vi "LSMcontroller_v56_from here for labview64bit.vi"() -> ()   [LabVIEW 2015] (continued)
                    n4222 = Bundle By Name(cluster=w1106, "Drawing Mode"=w1079, "measpoints"=w1095, "tt_cycles"=w1097, "refreshbuffer"=w1092, "refreshrate"=w1091, "Vx-ref"=w1098, "Vy-ref"=w1100, "srate"=w1089, "finite"=w1102, "cont"=w1101, "wavdet"=w1103, "avpp"=w1099, "srateAODO"=w1096, "bufferAI"=w1092, "bin"=w1094, "Angle Img"=w1086, "Vxminref"=w1085, "Vxmaxref"=w1084, "Vyminref"=w1083, "Vymaxref"=w1082, "Xpixels Img"=w1081, "Ypixels Img"=w1080, "Pel"=w1078, "Vz-reset"=0.0, "AIoverride"=w1076, "type"="Lifetime (contour)") -> (w1104:T12)
                    n4223 = Reciprocal(x=w1091) -> (1/x=w1088:dbl)
                    n4224 = local write "refreshtime"(w1088) -> ()
                    n4225 = call "2pparameters.vi"("Params in"=w1104, "command"="set") -> ()  [unwired: 1 out]
                  }
                  frame "X-Y-Z-t movie" {
                  }
                  frame "linescan" {
                  }
                  frame "Timetrace" {
                    n4226 = local read "Vy-min draw"() -> (w1116:dbl)
                    n4227 = local read "Vy-max draw"() -> (w1115:dbl)
                    n4228 = local read "Vx-min draw"() -> (w1118:dbl)
                    n4229 = local read "Vx-max draw"() -> (w1117:dbl)
                    n4230 = local read "xpixels ref"() -> (w1114:i32)
                    n4231 = local read "ypixels ref"() -> (w1113:i32)
                    n4232 = local read "ROI Type"() -> (w1112:u16)
                    n4233 = local read "srateAODOtt"() -> (w1123:dbl)
                    n4234 = local read "# of frames"() -> (w1128:i32)
                    n4235 = local read "refreshtime"() -> (w1120:dbl)
                    n4236 = local read "Pel"() -> (w1111:dbl)
                    n4237 = local read "bin"() -> (w1126:dbl)
                    n4238 = local read "Override AI buffer"() -> (w1109:bool)
                    n4239 = local read "finite samples"() -> (w1135:bool)
                    n4240 = local read "srateAODOtt"() -> (w1122:dbl)
                    n4241 = local read "srateAODOtt"() -> (w1129:dbl)
                    n4242 = local read "continuous"() -> (w1134:bool)
                    n4243 = local read "Angle ref"() -> (w1119:dbl)
                    n4244 = local read "wavdet"() -> (w1136:bool)
                    n4245 = local read "Vx-ref"() -> (w1131:dbl)
                    n4246 = local read "Vy-ref"() -> (w1133:dbl)
                    n4247 = local read "avpp"() -> (w1132:i32)
                    n4248 = call "tt_timeandsamples.vi"("bin"=w1126, "refreshtime"=w1120, "srateAODOtt"=w1123, "tot#ofsamples"=w1128) -> ("refreshrate"=w1124:dbl, "refreshbuffer"=w1125:i32, "timetracecycles"=w1130:i32)  [unwired: 5 in]
                    n4249 = local read "bin"() -> (w1127:dbl)
                    n4250 = call "2pparameters.vi"("command"="get") -> ("params out"=w1139:T12)  [unwired: 1 in]
                    n4251 = Bundle By Name(cluster=w1139, "Drawing Mode"=w1112, "measpoints"=w1128, "tt_cycles"=w1130, "refreshbuffer"=w1125, "refreshrate"=w1124, "Vx-ref"=w1131, "Vy-ref"=w1133, "srate"=w1122, "finite"=w1135, "cont"=w1134, "wavdet"=w1136, "avpp"=w1132, "srateAODO"=w1129, "bufferAI"=w1125, "bin"=w1127, "Angle Img"=w1119, "Vxminref"=w1118, "Vxmaxref"=w1117, "Vyminref"=w1116, "Vymaxref"=w1115, "Xpixels Img"=w1114, "Ypixels Img"=w1113, "Pel"=w1111, "Vz-reset"=0.0, "AIoverride"=w1109, "type"="Timetrace") -> (w1137:T12)
                    n4252 = Reciprocal(x=w1124) -> (1/x=w1121:dbl)
                    n4253 = local write "refreshtime"(w1121) -> ()
                    n4254 = call "2pparameters.vi"("Params in"=w1137, "command"="set") -> ()  [unwired: 1 out]
                  }
                  frame "Lifetime (point)" {
                  }
                }
              }
              frame #1 {
                w1142 = FALSE ("wavdet")
                n4255 = call "2pparameters.vi"("command"="get") -> ("params out"=w1146:T12)  [unwired: 1 in]
                n4256 = Bundle By Name(cluster=w1146, "finite"=w1142, "cont"=w1142, "wavdet"=TRUE) -> (w1143:T12)
                n4257 = call "2pparameters.vi"("Params in"=w1143, "command"="set") -> ()  [unwired: 1 out]
              }
              frame #2 {
                n4258 = local read "Meastab"() -> (w1151:enum32{"X-Y Image", "Linescan", "Timetrace"})
                n4259 = property on="refwf" class="Ring (strict)"() -> ("RingText.Text"=w1154:string)  [unwired: 2 in, 2 out]
                n4260 = case shown="\"Timetrace\"" w1151 {
                  tunnel: [w1164 w1165] -> w1150
                  frame "X-Y Image", Default {
                    n4261 = local read "Sampling rate"() -> (w1164:dbl)
                  }
                  frame "Timetrace" {
                    n4262 = local read "srateAODOtt"() -> (w1165:dbl)
                  }
                }
                n4263 = call "waveformsAObuffer.vi"("command"="get") -> ("AO wf out"=w1163:waveform(dbl)[])  [unwired: 1 in]
                n4264 = local read "wavdet"() -> (w1153:bool)
                n4265 = call "waveformsDObuffer.vi"("command"="get") -> ("DO wf out"=w1159:digitalwaveform[])  [unwired: 1 in]
                n4266 = call "correctwaveformsizetemp.vi"("new sampling frequency (Hz)"=w1150, "start"=FALSE, "reference waveforms to"=w1154, "Analog waveforms in"=w1163, "stop"=FALSE, "Digital waveforms in"=w1159) -> ("analog wf out"=w1157:waveform(dbl)[], "Digital wf out"=w1155:digitalwaveform[], "measpoints"=w1152:i32)
                n4267 = local write "Analog Lines Plot"(w1157) -> ()
                n4268 = call "GetNumCamFramesv2.vi"("Digital Waveform Graph"=w1155) -> ("Numeric"=w1156:i32)  [unwired: 10 in]
                n4269 = local write "Digital Lines Plot"(w1155) -> ()
                n4270 = call "waveformsDObuffer.vi"("DO wf in"=w1155, "command"="set") -> ()  [unwired: 1 out]
                n4271 = call "waveformsAObuffer.vi"("AO wf in"=w1157, "command"="set") -> ()  [unwired: 1 out]
                n4272 = local write "Total Camera Frames"(w1156) -> ()
                n4273 = case shown="True" w1153 {
                  tunnel: w1152 -> [_ w1166]
                  frame False {
                  }
                  frame True {
                    n4274 = local write "# of frames"(w1166) -> ()
                  }
                }
              }
              frame #3 {
                n4275 = local read "finite samples"() -> (w1167:bool)
                n4276 = local read "continuous"() -> (w1168:bool)
                n4277 = local read "wavdet"() -> (w1169:bool)
                n4278 = call "2pparameters.vi"("command"="get") -> ("params out"=w1172:T12)  [unwired: 1 in]
                n4279 = Bundle By Name(cluster=w1172, "finite"=w1167, "cont"=w1168, "wavdet"=w1169) -> (w1170:T12)
                n4280 = call "2pparameters.vi"("Params in"=w1170, "command"="set") -> ()  [unwired: 1 out]
              }
            }
          }
          event "Start amplitude (V)", "Cycles", "Baseline (V)", "Step size (V)", "DC (%)", "Period (ms)", "Repeats", "Pulses", "phase shift (ms)": Value Change {
            n4281 = event-data() -> ()  [unwired: 1 in, 6 out]
            n4282 = stacked-sequence {
              seq-local: [_ _ w1280 _ _] -> [_ _ _ w1302 _]
              seq-local: [_ _ w1279 _ _] -> [_ _ _ w1301 _]
              frame #0 {
                n4283 = local read "Measurement"() -> (w1174:T5)
                n4284 = case shown="\"X-Y-t movie\", Default" w1174 {
                  frame "X-Y-t movie", Default {
                    n4285 = local read "avpp"() -> (w1195:i32)
                    n4286 = local read "Angle ref"() -> (w1194:dbl)
                    n4287 = local read "ROI Type"() -> (w1193:u16)
                    n4288 = local read "xpixels ref"() -> (w1190:i32)
                    n4289 = local read "Vx-min ref"() -> (w1189:dbl)
                    n4290 = local read "Vx-max ref"() -> (w1188:dbl)
                    n4291 = local read "ypixels ref"() -> (w1186:i32)
                    n4292 = local read "Vy-min ref"() -> (w1187:dbl)
                    n4293 = local read "Vy-max ref"() -> (w1183:dbl)
                    n4294 = local read "Sampling rate"() -> (w1177:dbl)
                    n4295 = local read "finite samples"() -> (w1178:bool)
                    n4296 = local read "continuous"() -> (w1181:bool)
                    n4297 = local read "wavdet"() -> (w1182:bool)
                    n4298 = local read "# of frames"() -> (w1180:i32)
                    n4299 = local read "maxbufferAI"() -> (w1179:i32)
                    n4300 = local read "Override AI buffer"() -> (w1175:bool)
                    n4301 = call "2pparameters.vi"("command"="get") -> ("params out"=w1192:T12)  [unwired: 1 in]
                    n4302 = Bundle By Name(cluster=w1192, "type"="X-Y-t movie", "avpp"=w1195, "Angle Img"=w1194, "Xpixels Img"=w1190, "Vx-min Img"=w1189, "VX-max Img"=w1188, "Ypixels Img"=w1186, "Vy-min Img"=w1187, "Vy-max Img"=w1183, "srate"=w1177, "srate Img"=w1177, "finite"=w1178, "cont"=w1181, "wavdet"=w1182, "measpoints"=w1180, "maxbufferAI"=w1179, "Drawing Mode"=w1193, "Vz-reset"=0.0, "AIoverride"=w1175) -> (w1184:T12)
                    n4303 = call "2pparameters.vi"("Params in"=w1184, "command"="set") -> ()  [unwired: 1 out]
                  }
                  frame "X-Y-Z stack" {
                    n4304 = call "2pparameters.vi"("command"="get") -> ("params out"=w1199:T12)  [unwired: 1 in]
                    n4305 = Bundle By Name(cluster=w1199, "type"="X-Y-Z stack") -> (w1197:T12)
                    n4306 = call "2pparameters.vi"("Params in"=w1197, "command"="set") -> ()  [unwired: 1 out]
                  }
                  frame "Lifetime (scan)" {
                    n4307 = call "2pparameters.vi"("command"="get") -> ("params out"=w1204:T12)  [unwired: 1 in]
                    n4308 = Bundle By Name(cluster=w1204, "type"="Lifetime (scan)") -> (w1202:T12)
                    n4309 = call "2pparameters.vi"("Params in"=w1202, "command"="set") -> ()  [unwired: 1 out]
                  }
                  frame "Lifetime (contour)" {
                    n4310 = local read "Vy-min draw"() -> (w1214:dbl)
                    n4311 = local read "Vy-max draw"() -> (w1213:dbl)
                    n4312 = local read "Vx-min draw"() -> (w1216:dbl)
                    n4313 = local read "Vx-max draw"() -> (w1215:dbl)
                    n4314 = local read "xpixels ref"() -> (w1212:i32)
                    n4315 = local read "ypixels ref"() -> (w1211:i32)
                    n4316 = local read "ROI Type"() -> (w1210:u16)
                    n4317 = local read "srateAODOtt"() -> (w1221:dbl)
                    n4318 = local read "# of frames"() -> (w1226:i32)
                    n4319 = local read "refreshtime"() -> (w1218:dbl)
                    n4320 = local read "Pel"() -> (w1209:dbl)
                    n4321 = local read "bin"() -> (w1224:dbl)
                    n4322 = local read "Override AI buffer"() -> (w1207:bool)
                    n4323 = local read "finite samples"() -> (w1233:bool)
                    n4324 = local read "srateAODOtt"() -> (w1220:dbl)
                    n4325 = local read "srateAODOtt"() -> (w1227:dbl)
                    n4326 = local read "continuous"() -> (w1232:bool)
                    n4327 = local read "Angle ref"() -> (w1217:dbl)
                    n4328 = local read "wavdet"() -> (w1234:bool)
                    n4329 = local read "Vx-ref"() -> (w1229:dbl)
                    n4330 = local read "Vy-ref"() -> (w1231:dbl)
                    n4331 = local read "avpp"() -> (w1230:i32)
                    n4332 = call "tt_timeandsamples.vi"("bin"=w1224, "refreshtime"=w1218, "srateAODOtt"=w1221, "tot#ofsamples"=w1226) -> ("refreshrate"=w1222:dbl, "refreshbuffer"=w1223:i32, "timetracecycles"=w1228:i32)  [unwired: 5 in]
                    n4333 = local read "bin"() -> (w1225:dbl)
                    n4334 = call "2pparameters.vi"("command"="get") -> ("params out"=w1237:T12)  [unwired: 1 in]
                    n4335 = Bundle By Name(cluster=w1237, "Drawing Mode"=w1210, "measpoints"=w1226, "tt_cycles"=w1228, "refreshbuffer"=w1223, "refreshrate"=w1222, "Vx-ref"=w1229, "Vy-ref"=w1231, "srate"=w1220, "finite"=w1233, "cont"=w1232, "wavdet"=w1234, "avpp"=w1230, "srateAODO"=w1227, "bufferAI"=w1223, "bin"=w1225, "Angle Img"=w1217, "Vxminref"=w1216, "Vxmaxref"=w1215, "Vyminref"=w1214, "Vymaxref"=w1213, "Xpixels Img"=w1212, "Ypixels Img"=w1211, "Pel"=w1209, "Vz-reset"=0.0, "AIoverride"=w1207, "type"="Lifetime (contour)") -> (w1235:T12)
                    n4336 = Reciprocal(x=w1222) -> (1/x=w1219:dbl)
                    n4337 = local write "refreshtime"(w1219) -> ()
                    n4338 = call "2pparameters.vi"("Params in"=w1235, "command"="set") -> ()  [unwired: 1 out]
                  }
                  frame "X-Y-Z-t movie" {
                  }
                  frame "linescan" {
                  }
                  frame "Timetrace" {
                    n4339 = local read "Vy-min draw"() -> (w1247:dbl)
                    n4340 = local read "Vy-max draw"() -> (w1246:dbl)
                    n4341 = local read "Vx-min draw"() -> (w1249:dbl)
                    n4342 = local read "Vx-max draw"() -> (w1248:dbl)
                    n4343 = local read "xpixels ref"() -> (w1245:i32)
                    n4344 = local read "ypixels ref"() -> (w1244:i32)
                    n4345 = local read "ROI Type"() -> (w1243:u16)
                    n4346 = local read "srateAODOtt"() -> (w1254:dbl)
                    n4347 = local read "# of frames"() -> (w1259:i32)
                    n4348 = local read "refreshtime"() -> (w1251:dbl)
                    n4349 = local read "Pel"() -> (w1242:dbl)
                    n4350 = local read "bin"() -> (w1257:dbl)
                    n4351 = local read "Override AI buffer"() -> (w1240:bool)
                    n4352 = local read "finite samples"() -> (w1266:bool)
                    n4353 = local read "srateAODOtt"() -> (w1253:dbl)
                    n4354 = local read "srateAODOtt"() -> (w1260:dbl)
                    n4355 = local read "continuous"() -> (w1265:bool)
                    n4356 = local read "Angle ref"() -> (w1250:dbl)
                    n4357 = local read "wavdet"() -> (w1267:bool)
                    n4358 = local read "Vx-ref"() -> (w1262:dbl)
                    n4359 = local read "Vy-ref"() -> (w1264:dbl)
                    n4360 = local read "avpp"() -> (w1263:i32)
                    n4361 = call "tt_timeandsamples.vi"("bin"=w1257, "refreshtime"=w1251, "srateAODOtt"=w1254, "tot#ofsamples"=w1259) -> ("refreshrate"=w1255:dbl, "refreshbuffer"=w1256:i32, "timetracecycles"=w1261:i32)  [unwired: 5 in]
                    n4362 = local read "bin"() -> (w1258:dbl)
                    n4363 = call "2pparameters.vi"("command"="get") -> ("params out"=w1270:T12)  [unwired: 1 in]
                    n4364 = Bundle By Name(cluster=w1270, "Drawing Mode"=w1243, "measpoints"=w1259, "tt_cycles"=w1261, "refreshbuffer"=w1256, "refreshrate"=w1255, "Vx-ref"=w1262, "Vy-ref"=w1264, "srate"=w1253, "finite"=w1266, "cont"=w1265, "wavdet"=w1267, "avpp"=w1263, "srateAODO"=w1260, "bufferAI"=w1256, "bin"=w1258, "Angle Img"=w1250, "Vxminref"=w1249, "Vxmaxref"=w1248, "Vyminref"=w1247, "Vymaxref"=w1246, "Xpixels Img"=w1245, "Ypixels Img"=w1244, "Pel"=w1242, "Vz-reset"=0.0, "AIoverride"=w1240, "type"="Timetrace") -> (w1268:T12)
                    n4365 = Reciprocal(x=w1255) -> (1/x=w1252:dbl)
                    n4366 = local write "refreshtime"(w1252) -> ()
                    n4367 = call "2pparameters.vi"("Params in"=w1268, "command"="set") -> ()  [unwired: 1 out]
                  }
                  frame "Lifetime (point)" {
                  }
                }
              }
              frame #1 {
                w1273 = FALSE ("wavdet")
                n4368 = call "2pparameters.vi"("command"="get") -> ("params out"=w1277:T12)  [unwired: 1 in]
                n4369 = Bundle By Name(cluster=w1277, "finite"=w1273, "cont"=w1273, "wavdet"=TRUE) -> (w1274:T12)
                n4370 = call "2pparameters.vi"("Params in"=w1274, "command"="set") -> ()  [unwired: 1 out]
              }
              frame #2 {
                n4371 = local read "AO channels"() -> (w1282:u32)
                n4372 = call "2pparameters.vi"("command"="get") -> ("params out"=w1284:T12)  [unwired: 1 in]
                n4373 = Unbundle By Name(w1284) -> ("aAO"=w1283:u32[])
                n4374 = Search 1D Array(1D array=w1283, element=w1282) -> (index of element=w1280:i32)  [unwired: 1 in]
                n4375 = Greater?(x=w1280, y=-1) -> (0:w1279:bool)
                n4376 = case shown="True" w1279 {
                  tunnel: w1280 -> [_ w1298]
                  frame False {
                  }
                  frame True {
                    n4377 = local read "Meastab"() -> (w1287:enum32{"X-Y Image", "Linescan", "Timetrace"})
                    n4378 = case shown="\"Timetrace\"" w1287 {
                      tunnel: [w1299 w1300] -> w1286
                      frame "X-Y Image", Default {
                        n4379 = local read "Sampling rate"() -> (w1299:dbl)
                      }
                      frame "Timetrace" {
                        n4380 = local read "srateAODOtt"() -> (w1300:dbl)
                      }
                    }
                    n4381 = local read "Start amplitude (V)"() -> (w1295:dbl)
                    n4382 = local read "phase shift (ms)"() -> (w1290:dbl)
                    n4383 = local read "Step size (V)"() -> (w1293:dbl)
                    n4384 = local read "Baseline (V)"() -> (w1294:dbl)
                    n4385 = local read "Period (ms)"() -> (w1291:dbl)
                    n4386 = local read "padding value"() -> (w1288:dbl)
                    n4387 = local read "Repeats"() -> (w1297:dbl)
                    n4388 = local read "Cycles"() -> (w1296:dbl)
                    n4389 = local read "DC (%)"() -> (w1292:dbl)
                    n4390 = local read "Pulses"() -> (w1289:dbl)
                    n4391 = call "replace AO square wf param.vi"("Baseline (V)"=w1294, "Start amplitude (V)"=w1295, "Cycles"=w1296, "Repeats"=w1297, "index of AO wave"=w1298, "Step size (V)"=w1293, "DC (%)"=w1292, "Sampling frequency (Hz)"=w1286, "Period (ms)"=w1291, "Cycle length (s)"=w1290, "Pulses"=w1289, "padding value"=w1288) -> ()  [unwired: 4 in]
                  }
                }
              }
              frame #3 {
                n4392 = case shown="True" w1301 {
                  tunnel: w1302 -> [_ w1310]
                  frame False {
                  }
                  frame True {
                    n4393 = call "waveformparamsv2.vi"("command"="get") -> ("Params out"=w1324:T16)  [unwired: 4 in, 2 out]
                    n4394 = Unbundle By Name(w1324) -> ("AO parameters"=w1323:T17)
                    n4395 = local read "Meastab"() -> (w1305:enum32{"X-Y Image", "Linescan", "Timetrace"})
                    n4396 = case shown="\"Timetrace\"" w1305 {
                      tunnel: [w1326 w1327] -> w1314
                      frame "X-Y Image", Default {
                        n4397 = local read "Sampling rate"() -> (w1326:dbl)
                      }
                      frame "Timetrace" {
                        n4398 = local read "srateAODOtt"() -> (w1327:dbl)
                      }
                    }
                    n4399 = Index Array(array=w1323, index=w1310) -> (element=w1312:T18)
                    n4400 = call "waveformsAObuffer.vi"("command"="get") -> ("AO wf out"=w1311:waveform(dbl)[])  [unwired: 1 in]
                    n4401 = call "generateRampedSquareWave_fromAOparameters.vi"("AO params"=w1312) -> ("Waveform"=w1309:waveform(dbl))  [unwired: 1 out]
                    n4402 = property on="refwf" class="Ring (strict)"() -> ("RingText.Text"=w1313:string)  [unwired: 2 in, 2 out]
                    n4403 = Replace Array Subset(array=w1311, new element=w1309, index=w1310) -> (w1308:waveform(dbl)[])
                    n4404 = call "waveformsDObuffer.vi"("command"="get") -> ("DO wf out"=w1319:digitalwaveform[])  [unwired: 1 in]
                    n4405 = call "correctwaveformsizetemp.vi"("new sampling frequency (Hz)"=w1314, "start"=FALSE, "reference waveforms to"=w1313, "Analog waveforms in"=w1308, "stop"=FALSE, "Digital waveforms in"=w1319) -> ("analog wf out"=w1317:waveform(dbl)[], "Digital wf out"=w1315:digitalwaveform[], "measpoints"=w1306:i32)
                    n4406 = local read "wavdet"() -> (w1307:bool)
                    n4407 = local write "Analog Lines Plot"(w1317) -> ()
                    n4408 = call "GetNumCamFramesv2.vi"("Digital Waveform Graph"=w1315) -> ("Numeric"=w1316:i32)  [unwired: 10 in]
                    n4409 = local write "Digital Lines Plot"(w1315) -> ()
                    n4410 = call "waveformsAObuffer.vi"("AO wf in"=w1317, "command"="set") -> ()  [unwired: 1 out]
                    n4411 = call "waveformsDObuffer.vi"("DO wf in"=w1315, "command"="set") -> ()  [unwired: 1 out]
                    n4412 = local write "Total Camera Frames"(w1316) -> ()
                    n4413 = case shown="True" w1307 {
                      tunnel: w1306 -> [_ w1328]
                      frame False {
                      }
                      frame True {
                        n4414 = local write "# of frames"(w1328) -> ()
                      }
                    }
                  }
                }
              }
              frame #4 {
                n4415 = local read "finite samples"() -> (w1329:bool)
                n4416 = local read "continuous"() -> (w1330:bool)
                n4417 = local read "wavdet"() -> (w1331:bool)
                n4418 = call "2pparameters.vi"("command"="get") -> ("params out"=w1334:T12)  [unwired: 1 in]
                n4419 = Bundle By Name(cluster=w1334, "finite"=w1329, "cont"=w1330, "wavdet"=w1331) -> (w1332:T12)
                n4420 = call "2pparameters.vi"("Params in"=w1332, "command"="set") -> ()  [unwired: 1 out]
              }
            }
          }
          event "Amplitude (V)", "Offset (V)", "Frequency", "Tri Repeats": Value Change {
            n4421 = event-data() -> ()  [unwired: 1 in, 6 out]
            n4422 = stacked-sequence {
              seq-local: [_ _ w1442 _ _] -> [_ _ _ w1460 _]
              seq-local: [_ _ w1441 _ _] -> [_ _ _ w1459 _]
              frame #0 {
                n4423 = local read "Measurement"() -> (w1336:T5)
                n4424 = case shown="\"X-Y-t movie\", Default" w1336 {
                  frame "X-Y-t movie", Default {
                    n4425 = local read "avpp"() -> (w1357:i32)
                    n4426 = local read "Angle ref"() -> (w1356:dbl)
                    n4427 = local read "ROI Type"() -> (w1355:u16)
                    n4428 = local read "xpixels ref"() -> (w1352:i32)
                    n4429 = local read "Vx-min ref"() -> (w1351:dbl)
                    n4430 = local read "Vx-max ref"() -> (w1350:dbl)
                    n4431 = local read "ypixels ref"() -> (w1348:i32)
                    n4432 = local read "Vy-min ref"() -> (w1349:dbl)
                    n4433 = local read "Vy-max ref"() -> (w1345:dbl)
                    n4434 = local read "Sampling rate"() -> (w1339:dbl)
                    n4435 = local read "finite samples"() -> (w1340:bool)
                    n4436 = local read "continuous"() -> (w1343:bool)
                    n4437 = local read "wavdet"() -> (w1344:bool)
                    n4438 = local read "# of frames"() -> (w1342:i32)
                    n4439 = local read "maxbufferAI"() -> (w1341:i32)
                    n4440 = local read "Override AI buffer"() -> (w1337:bool)
                    n4441 = call "2pparameters.vi"("command"="get") -> ("params out"=w1354:T12)  [unwired: 1 in]
                    n4442 = Bundle By Name(cluster=w1354, "type"="X-Y-t movie", "avpp"=w1357, "Angle Img"=w1356, "Xpixels Img"=w1352, "Vx-min Img"=w1351, "VX-max Img"=w1350, "Ypixels Img"=w1348, "Vy-min Img"=w1349, "Vy-max Img"=w1345, "srate"=w1339, "srate Img"=w1339, "finite"=w1340, "cont"=w1343, "wavdet"=w1344, "measpoints"=w1342, "maxbufferAI"=w1341, "Drawing Mode"=w1355, "Vz-reset"=0.0, "AIoverride"=w1337) -> (w1346:T12)
                    n4443 = call "2pparameters.vi"("Params in"=w1346, "command"="set") -> ()  [unwired: 1 out]
                  }
                  frame "X-Y-Z stack" {
                    n4444 = call "2pparameters.vi"("command"="get") -> ("params out"=w1361:T12)  [unwired: 1 in]
                    n4445 = Bundle By Name(cluster=w1361, "type"="X-Y-Z stack") -> (w1359:T12)
                    n4446 = call "2pparameters.vi"("Params in"=w1359, "command"="set") -> ()  [unwired: 1 out]
                  }
                  frame "Lifetime (scan)" {
                    n4447 = call "2pparameters.vi"("command"="get") -> ("params out"=w1366:T12)  [unwired: 1 in]
                    n4448 = Bundle By Name(cluster=w1366, "type"="Lifetime (scan)") -> (w1364:T12)
                    n4449 = call "2pparameters.vi"("Params in"=w1364, "command"="set") -> ()  [unwired: 1 out]
                  }
                  frame "Lifetime (contour)" {
                    n4450 = local read "Vy-min draw"() -> (w1376:dbl)
                    n4451 = local read "Vy-max draw"() -> (w1375:dbl)
                    n4452 = local read "Vx-min draw"() -> (w1378:dbl)
                    n4453 = local read "Vx-max draw"() -> (w1377:dbl)
                    n4454 = local read "xpixels ref"() -> (w1374:i32)
                    n4455 = local read "ypixels ref"() -> (w1373:i32)
                    n4456 = local read "ROI Type"() -> (w1372:u16)
                    n4457 = local read "srateAODOtt"() -> (w1383:dbl)
                    n4458 = local read "# of frames"() -> (w1388:i32)
                    n4459 = local read "refreshtime"() -> (w1380:dbl)
                    n4460 = local read "Pel"() -> (w1371:dbl)
                    n4461 = local read "bin"() -> (w1386:dbl)
                    n4462 = local read "Override AI buffer"() -> (w1369:bool)
                    n4463 = local read "finite samples"() -> (w1395:bool)
                    n4464 = local read "srateAODOtt"() -> (w1382:dbl)
                    n4465 = local read "srateAODOtt"() -> (w1389:dbl)
                    n4466 = local read "continuous"() -> (w1394:bool)
                    n4467 = local read "Angle ref"() -> (w1379:dbl)
                    n4468 = local read "wavdet"() -> (w1396:bool)
                    n4469 = local read "Vx-ref"() -> (w1391:dbl)
                    n4470 = local read "Vy-ref"() -> (w1393:dbl)
                    n4471 = local read "avpp"() -> (w1392:i32)
                    n4472 = call "tt_timeandsamples.vi"("bin"=w1386, "refreshtime"=w1380, "srateAODOtt"=w1383, "tot#ofsamples"=w1388) -> ("refreshrate"=w1384:dbl, "refreshbuffer"=w1385:i32, "timetracecycles"=w1390:i32)  [unwired: 5 in]
                    n4473 = local read "bin"() -> (w1387:dbl)
                    n4474 = call "2pparameters.vi"("command"="get") -> ("params out"=w1399:T12)  [unwired: 1 in]
                    n4475 = Bundle By Name(cluster=w1399, "Drawing Mode"=w1372, "measpoints"=w1388, "tt_cycles"=w1390, "refreshbuffer"=w1385, "refreshrate"=w1384, "Vx-ref"=w1391, "Vy-ref"=w1393, "srate"=w1382, "finite"=w1395, "cont"=w1394, "wavdet"=w1396, "avpp"=w1392, "srateAODO"=w1389, "bufferAI"=w1385, "bin"=w1387, "Angle Img"=w1379, "Vxminref"=w1378, "Vxmaxref"=w1377, "Vyminref"=w1376, "Vymaxref"=w1375, "Xpixels Img"=w1374, "Ypixels Img"=w1373, "Pel"=w1371, "Vz-reset"=0.0, "AIoverride"=w1369, "type"="Lifetime (contour)") -> (w1397:T12)
                    n4476 = Reciprocal(x=w1384) -> (1/x=w1381:dbl)
                    n4477 = local write "refreshtime"(w1381) -> ()
                    n4478 = call "2pparameters.vi"("Params in"=w1397, "command"="set") -> ()  [unwired: 1 out]
                  }
                  frame "X-Y-Z-t movie" {
                  }
                  frame "linescan" {
                  }
                  frame "Timetrace" {
                    n4479 = local read "Vy-min draw"() -> (w1409:dbl)
                    n4480 = local read "Vy-max draw"() -> (w1408:dbl)
                    n4481 = local read "Vx-min draw"() -> (w1411:dbl)
                    n4482 = local read "Vx-max draw"() -> (w1410:dbl)
                    n4483 = local read "xpixels ref"() -> (w1407:i32)
                    n4484 = local read "ypixels ref"() -> (w1406:i32)
                    n4485 = local read "ROI Type"() -> (w1405:u16)
                    n4486 = local read "srateAODOtt"() -> (w1416:dbl)
                    n4487 = local read "# of frames"() -> (w1421:i32)
                    n4488 = local read "refreshtime"() -> (w1413:dbl)
                    n4489 = local read "Pel"() -> (w1404:dbl)
                    n4490 = local read "bin"() -> (w1419:dbl)
                    n4491 = local read "Override AI buffer"() -> (w1402:bool)
                    n4492 = local read "finite samples"() -> (w1428:bool)
                    n4493 = local read "srateAODOtt"() -> (w1415:dbl)
                    n4494 = local read "srateAODOtt"() -> (w1422:dbl)
                    n4495 = local read "continuous"() -> (w1427:bool)
                    n4496 = local read "Angle ref"() -> (w1412:dbl)
                    n4497 = local read "wavdet"() -> (w1429:bool)
                    n4498 = local read "Vx-ref"() -> (w1424:dbl)
                    n4499 = local read "Vy-ref"() -> (w1426:dbl)
                    n4500 = local read "avpp"() -> (w1425:i32)
                    n4501 = call "tt_timeandsamples.vi"("bin"=w1419, "refreshtime"=w1413, "srateAODOtt"=w1416, "tot#ofsamples"=w1421) -> ("refreshrate"=w1417:dbl, "refreshbuffer"=w1418:i32, "timetracecycles"=w1423:i32)  [unwired: 5 in]
                    n4502 = local read "bin"() -> (w1420:dbl)
                    n4503 = call "2pparameters.vi"("command"="get") -> ("params out"=w1432:T12)  [unwired: 1 in]
                    n4504 = Bundle By Name(cluster=w1432, "Drawing Mode"=w1405, "measpoints"=w1421, "tt_cycles"=w1423, "refreshbuffer"=w1418, "refreshrate"=w1417, "Vx-ref"=w1424, "Vy-ref"=w1426, "srate"=w1415, "finite"=w1428, "cont"=w1427, "wavdet"=w1429, "avpp"=w1425, "srateAODO"=w1422, "bufferAI"=w1418, "bin"=w1420, "Angle Img"=w1412, "Vxminref"=w1411, "Vxmaxref"=w1410, "Vyminref"=w1409, "Vymaxref"=w1408, "Xpixels Img"=w1407, "Ypixels Img"=w1406, "Pel"=w1404, "Vz-reset"=0.0, "AIoverride"=w1402, "type"="Timetrace") -> (w1430:T12)
                    n4505 = Reciprocal(x=w1417) -> (1/x=w1414:dbl)
                    n4506 = local write "refreshtime"(w1414) -> ()
                    n4507 = call "2pparameters.vi"("Params in"=w1430, "command"="set") -> ()  [unwired: 1 out]
                  }
                  frame "Lifetime (point)" {
                  }
                }
              }
              frame #1 {
                w1435 = FALSE ("wavdet")
                n4508 = call "2pparameters.vi"("command"="get") -> ("params out"=w1439:T12)  [unwired: 1 in]
                n4509 = Bundle By Name(cluster=w1439, "finite"=w1435, "cont"=w1435, "wavdet"=TRUE) -> (w1436:T12)
                n4510 = call "2pparameters.vi"("Params in"=w1436, "command"="set") -> ()  [unwired: 1 out]
              }
              frame #2 {
                n4511 = local read "AO channels"() -> (w1444:u32)
                n4512 = call "2pparameters.vi"("command"="get") -> ("params out"=w1446:T12)  [unwired: 1 in]
                n4513 = Unbundle By Name(w1446) -> ("aAO"=w1445:u32[])
                n4514 = Search 1D Array(1D array=w1445, element=w1444) -> (index of element=w1442:i32)  [unwired: 1 in]
                n4515 = Greater?(x=w1442, y=-1) -> (0:w1441:bool)
                n4516 = case shown="True" w1441 {
                  tunnel: w1442 -> [_ w1456]
                  frame False {
                  }
                  frame True {
                    n4517 = local read "Meastab"() -> (w1449:enum32{"X-Y Image", "Linescan", "Timetrace"})
                    n4518 = local read "Tri padding value"() -> (w1450:dbl)
                    n4519 = local read "Amplitude (V)"() -> (w1454:dbl)
                    n4520 = local read "Tri Phase (s)"() -> (w1451:dbl)
                    n4521 = local read "Tri Repeats"() -> (w1452:dbl)
                    n4522 = local read "Frequency"() -> (w1453:dbl)
                    n4523 = local read "Offset (V)"() -> (w1455:dbl)
                    n4524 = case shown="\"Timetrace\"" w1449 {
                      tunnel: [w1457 w1458] -> w1448
                      frame "X-Y Image", Default {
                        n4525 = local read "Sampling rate"() -> (w1457:dbl)
                      }
                      frame "Timetrace" {
                        n4526 = local read "srateAODOtt"() -> (w1458:dbl)
                      }
                    }
                    n4527 = call "replace AO tri wf param.vi"("padding value"=w1450, "index of AO wave"=w1456, "Tri phase"=w1451, "Sampling frequency (Hz)"=w1448, "Tri Repeats"=w1452, "Frequency"=w1453, "Amplitude (V)"=w1454, "Offset (V)"=w1455) -> ()
                  }
                }
              }
              frame #3 {
                n4528 = case shown="True" w1459 {
                  tunnel: w1460 -> [_ w1469]
                  frame False {
                  }
                  frame True {
                    n4529 = call "waveformparamsv2.vi"("command"="get") -> ("Params out"=w1482:T16)  [unwired: 4 in, 2 out]
                    n4530 = Unbundle By Name(w1482) -> ("AO parameters"=w1481:T17)
                    n4531 = local read "Meastab"() -> (w1464:enum32{"X-Y Image", "Linescan", "Timetrace"})
                    n4532 = case shown="\"Timetrace\"" w1464 {
                      tunnel: [w1484 w1485] -> w1463
                      frame "X-Y Image", Default {
                        n4533 = local read "Sampling rate"() -> (w1484:dbl)
                      }
                      frame "Timetrace" {
                        n4534 = local read "srateAODOtt"() -> (w1485:dbl)
                      }
                    }
                    n4535 = Index Array(array=w1481, index=w1469) -> (element=w1471:T18)
                    n4536 = call "waveformsAObuffer.vi"("command"="get") -> ("AO wf out"=w1470:waveform(dbl)[])  [unwired: 1 in]
                    n4537 = call "generateTriWave_fromAOparameters.vi"("AO params"=w1471) -> ("Waveform"=w1468:waveform(dbl))  [unwired: 1 out]
                    n4538 = property on="refwf" class="Ring (strict)"() -> ("RingText.Text"=w1472:string)  [unwired: 2 in, 2 out]
                    n4539 = Replace Array Subset(array=w1470, new element=w1468, index=w1469) -> (w1467:waveform(dbl)[])
                    n4540 = call "waveformsDObuffer.vi"("command"="get") -> ("DO wf out"=w1477:digitalwaveform[])  [unwired: 1 in]
                    n4541 = call "correctwaveformsizetemp.vi"("new sampling frequency (Hz)"=w1463, "start"=FALSE, "reference waveforms to"=w1472, "Analog waveforms in"=w1467, "stop"=FALSE, "Digital waveforms in"=w1477) -> ("analog wf out"=w1475:waveform(dbl)[], "Digital wf out"=w1473:digitalwaveform[], "measpoints"=w1465:i32)
                    n4542 = local read "wavdet"() -> (w1466:bool)
                    n4543 = local write "Analog Lines Plot"(w1475) -> ()
                    n4544 = call "GetNumCamFramesv2.vi"("Digital Waveform Graph"=w1473) -> ("Numeric"=w1474:i32)  [unwired: 10 in]
                    n4545 = local write "Digital Lines Plot"(w1473) -> ()
                    n4546 = call "waveformsAObuffer.vi"("AO wf in"=w1475, "command"="set") -> ()  [unwired: 1 out]
                    n4547 = call "waveformsDObuffer.vi"("DO wf in"=w1473, "command"="set") -> ()  [unwired: 1 out]
                    n4548 = local write "Total Camera Frames"(w1474) -> ()
                    n4549 = case shown="True" w1466 {
                      tunnel: w1465 -> [_ w1486]
                      frame False {
                      }
                      frame True {
                        n4550 = local write "# of frames"(w1486) -> ()
                      }
                    }
                  }
                }
              }
              frame #4 {
                n4551 = local read "finite samples"() -> (w1487:bool)
                n4552 = local read "continuous"() -> (w1488:bool)
                n4553 = local read "wavdet"() -> (w1489:bool)
                n4554 = call "2pparameters.vi"("command"="get") -> ("params out"=w1492:T12)  [unwired: 1 in]
                n4555 = Bundle By Name(cluster=w1492, "finite"=w1487, "cont"=w1488, "wavdet"=w1489) -> (w1490:T12)
                n4556 = call "2pparameters.vi"("Params in"=w1490, "command"="set") -> ()  [unwired: 1 out]
              }
            }
          }
          event "Load Matlab Waveform": Value Change {
            n4557 = event-data() -> ()  [unwired: 1 in, 6 out]
            n4558 = stacked-sequence {
              seq-local: [_ _ w1600 _ _] -> [_ _ _ w1615 _]
              seq-local: [_ _ w1599 _ _] -> [_ _ _ w1614 _]
              frame #0 {
                n4559 = local read "Measurement"() -> (w1494:T5)
                n4560 = case shown="\"X-Y-t movie\", Default" w1494 {
                  frame "X-Y-t movie", Default {
                    n4561 = local read "avpp"() -> (w1515:i32)
                    n4562 = local read "Angle ref"() -> (w1514:dbl)
                    n4563 = local read "ROI Type"() -> (w1513:u16)
                    n4564 = local read "xpixels ref"() -> (w1510:i32)
                    n4565 = local read "Vx-min ref"() -> (w1509:dbl)
                    n4566 = local read "Vx-max ref"() -> (w1508:dbl)
                    n4567 = local read "ypixels ref"() -> (w1506:i32)
                    n4568 = local read "Vy-min ref"() -> (w1507:dbl)
                    n4569 = local read "Vy-max ref"() -> (w1503:dbl)
                    n4570 = local read "Sampling rate"() -> (w1497:dbl)
                    n4571 = local read "finite samples"() -> (w1498:bool)
                    n4572 = local read "continuous"() -> (w1501:bool)
                    n4573 = local read "wavdet"() -> (w1502:bool)
                    n4574 = local read "# of frames"() -> (w1500:i32)
                    n4575 = local read "maxbufferAI"() -> (w1499:i32)
                    n4576 = local read "Override AI buffer"() -> (w1495:bool)
                    n4577 = call "2pparameters.vi"("command"="get") -> ("params out"=w1512:T12)  [unwired: 1 in]
                    n4578 = Bundle By Name(cluster=w1512, "type"="X-Y-t movie", "avpp"=w1515, "Angle Img"=w1514, "Xpixels Img"=w1510, "Vx-min Img"=w1509, "VX-max Img"=w1508, "Ypixels Img"=w1506, "Vy-min Img"=w1507, "Vy-max Img"=w1503, "srate"=w1497, "srate Img"=w1497, "finite"=w1498, "cont"=w1501, "wavdet"=w1502, "measpoints"=w1500, "maxbufferAI"=w1499, "Drawing Mode"=w1513, "Vz-reset"=0.0, "AIoverride"=w1495) -> (w1504:T12)
                    n4579 = call "2pparameters.vi"("Params in"=w1504, "command"="set") -> ()  [unwired: 1 out]
                  }
                  frame "X-Y-Z stack" {
                    n4580 = call "2pparameters.vi"("command"="get") -> ("params out"=w1519:T12)  [unwired: 1 in]
                    n4581 = Bundle By Name(cluster=w1519, "type"="X-Y-Z stack") -> (w1517:T12)
                    n4582 = call "2pparameters.vi"("Params in"=w1517, "command"="set") -> ()  [unwired: 1 out]
                  }
                  frame "Lifetime (scan)" {
                    n4583 = call "2pparameters.vi"("command"="get") -> ("params out"=w1524:T12)  [unwired: 1 in]
                    n4584 = Bundle By Name(cluster=w1524, "type"="Lifetime (scan)") -> (w1522:T12)
                    n4585 = call "2pparameters.vi"("Params in"=w1522, "command"="set") -> ()  [unwired: 1 out]
                  }
                  frame "Lifetime (contour)" {
                    n4586 = local read "Vy-min draw"() -> (w1534:dbl)
                    n4587 = local read "Vy-max draw"() -> (w1533:dbl)
                    n4588 = local read "Vx-min draw"() -> (w1536:dbl)
                    n4589 = local read "Vx-max draw"() -> (w1535:dbl)
                    n4590 = local read "xpixels ref"() -> (w1532:i32)
                    n4591 = local read "ypixels ref"() -> (w1531:i32)
                    n4592 = local read "ROI Type"() -> (w1530:u16)
                    n4593 = local read "srateAODOtt"() -> (w1541:dbl)
                    n4594 = local read "# of frames"() -> (w1546:i32)
                    n4595 = local read "refreshtime"() -> (w1538:dbl)
                    n4596 = local read "Pel"() -> (w1529:dbl)
                    n4597 = local read "bin"() -> (w1544:dbl)
                    n4598 = local read "Override AI buffer"() -> (w1527:bool)
                    n4599 = local read "finite samples"() -> (w1553:bool)
                    n4600 = local read "srateAODOtt"() -> (w1540:dbl)
                    n4601 = local read "srateAODOtt"() -> (w1547:dbl)
                    n4602 = local read "continuous"() -> (w1552:bool)
                    n4603 = local read "Angle ref"() -> (w1537:dbl)
                    n4604 = local read "wavdet"() -> (w1554:bool)
                    n4605 = local read "Vx-ref"() -> (w1549:dbl)
                    n4606 = local read "Vy-ref"() -> (w1551:dbl)
                    n4607 = local read "avpp"() -> (w1550:i32)
                    n4608 = call "tt_timeandsamples.vi"("bin"=w1544, "refreshtime"=w1538, "srateAODOtt"=w1541, "tot#ofsamples"=w1546) -> ("refreshrate"=w1542:dbl, "refreshbuffer"=w1543:i32, "timetracecycles"=w1548:i32)  [unwired: 5 in]
                    n4609 = local read "bin"() -> (w1545:dbl)
                    n4610 = call "2pparameters.vi"("command"="get") -> ("params out"=w1557:T12)  [unwired: 1 in]
                    n4611 = Bundle By Name(cluster=w1557, "Drawing Mode"=w1530, "measpoints"=w1546, "tt_cycles"=w1548, "refreshbuffer"=w1543, "refreshrate"=w1542, "Vx-ref"=w1549, "Vy-ref"=w1551, "srate"=w1540, "finite"=w1553, "cont"=w1552, "wavdet"=w1554, "avpp"=w1550, "srateAODO"=w1547, "bufferAI"=w1543, "bin"=w1545, "Angle Img"=w1537, "Vxminref"=w1536, "Vxmaxref"=w1535, "Vyminref"=w1534, "Vymaxref"=w1533, "Xpixels Img"=w1532, "Ypixels Img"=w1531, "Pel"=w1529, "Vz-reset"=0.0, "AIoverride"=w1527, "type"="Lifetime (contour)") -> (w1555:T12)
                    n4612 = Reciprocal(x=w1542) -> (1/x=w1539:dbl)
                    n4613 = local write "refreshtime"(w1539) -> ()
                    n4614 = call "2pparameters.vi"("Params in"=w1555, "command"="set") -> ()  [unwired: 1 out]
                  }
                  frame "X-Y-Z-t movie" {
                  }
                  frame "linescan" {
                  }
                  frame "Timetrace" {
                    n4615 = local read "Vy-min draw"() -> (w1567:dbl)
                    n4616 = local read "Vy-max draw"() -> (w1566:dbl)
                    n4617 = local read "Vx-min draw"() -> (w1569:dbl)
                    n4618 = local read "Vx-max draw"() -> (w1568:dbl)
                    n4619 = local read "xpixels ref"() -> (w1565:i32)
                    n4620 = local read "ypixels ref"() -> (w1564:i32)
                    n4621 = local read "ROI Type"() -> (w1563:u16)
                    n4622 = local read "srateAODOtt"() -> (w1574:dbl)
                    n4623 = local read "# of frames"() -> (w1579:i32)
                    n4624 = local read "refreshtime"() -> (w1571:dbl)
                    n4625 = local read "Pel"() -> (w1562:dbl)
                    n4626 = local read "bin"() -> (w1577:dbl)
                    n4627 = local read "Override AI buffer"() -> (w1560:bool)
                    n4628 = local read "finite samples"() -> (w1586:bool)
                    n4629 = local read "srateAODOtt"() -> (w1573:dbl)
                    n4630 = local read "srateAODOtt"() -> (w1580:dbl)
                    n4631 = local read "continuous"() -> (w1585:bool)
                    n4632 = local read "Angle ref"() -> (w1570:dbl)
                    n4633 = local read "wavdet"() -> (w1587:bool)
                    n4634 = local read "Vx-ref"() -> (w1582:dbl)
                    n4635 = local read "Vy-ref"() -> (w1584:dbl)
                    n4636 = local read "avpp"() -> (w1583:i32)
                    n4637 = call "tt_timeandsamples.vi"("bin"=w1577, "refreshtime"=w1571, "srateAODOtt"=w1574, "tot#ofsamples"=w1579) -> ("refreshrate"=w1575:dbl, "refreshbuffer"=w1576:i32, "timetracecycles"=w1581:i32)  [unwired: 5 in]
                    n4638 = local read "bin"() -> (w1578:dbl)
                    n4639 = call "2pparameters.vi"("command"="get") -> ("params out"=w1590:T12)  [unwired: 1 in]
                    n4640 = Bundle By Name(cluster=w1590, "Drawing Mode"=w1563, "measpoints"=w1579, "tt_cycles"=w1581, "refreshbuffer"=w1576, "refreshrate"=w1575, "Vx-ref"=w1582, "Vy-ref"=w1584, "srate"=w1573, "finite"=w1586, "cont"=w1585, "wavdet"=w1587, "avpp"=w1583, "srateAODO"=w1580, "bufferAI"=w1576, "bin"=w1578, "Angle Img"=w1570, "Vxminref"=w1569, "Vxmaxref"=w1568, "Vyminref"=w1567, "Vymaxref"=w1566, "Xpixels Img"=w1565, "Ypixels Img"=w1564, "Pel"=w1562, "Vz-reset"=0.0, "AIoverride"=w1560, "type"="Timetrace") -> (w1588:T12)
                    n4641 = Reciprocal(x=w1575) -> (1/x=w1572:dbl)
                    n4642 = local write "refreshtime"(w1572) -> ()
                    n4643 = call "2pparameters.vi"("Params in"=w1588, "command"="set") -> ()  [unwired: 1 out]
                  }
                  frame "Lifetime (point)" {
                  }
                }
              }
              frame #1 {
                w1593 = FALSE ("wavdet")
                n4644 = call "2pparameters.vi"("command"="get") -> ("params out"=w1597:T12)  [unwired: 1 in]
                n4645 = Bundle By Name(cluster=w1597, "finite"=w1593, "cont"=w1593, "wavdet"=TRUE) -> (w1594:T12)
                n4646 = call "2pparameters.vi"("Params in"=w1594, "command"="set") -> ()  [unwired: 1 out]
              }
              frame #2 {
                n4647 = local read "AO channels"() -> (w1602:u32)
                n4648 = call "2pparameters.vi"("command"="get") -> ("params out"=w1604:T12)  [unwired: 1 in]
                n4649 = Unbundle By Name(w1604) -> ("aAO"=w1603:u32[])
                n4650 = Search 1D Array(1D array=w1603, element=w1602) -> (index of element=w1600:i32)  [unwired: 1 in]
                n4651 = Greater?(x=w1600, y=-1) -> (0:w1599:bool)
                n4652 = case shown="True" w1599 {
                  tunnel: w1600 -> [_ w1611]
                  frame False {
                  }
                  frame True {
                    n4653 = local read "Meastab"() -> (w1607:enum32{"X-Y Image", "Linescan", "Timetrace"})
                    n4654 = local read "Matlab waveform path"() -> (w1609:path)
                    n4655 = local read "Matlab padding value"() -> (w1610:dbl)
                    n4656 = case shown="\"Timetrace\"" w1607 {
                      tunnel: [w1612 w1613] -> w1606
                      frame "X-Y Image", Default {
                        n4657 = local read "Sampling rate"() -> (w1612:dbl)
                      }
                      frame "Timetrace" {
                        n4658 = local read "srateAODOtt"() -> (w1613:dbl)
                      }
                    }
                    n4659 = call "matlabwfexistsdialogue.vi"("Matlab waveform path"=w1609) -> ("mtalab waveform path out"=w1608:path)
                    n4660 = call "replace AO matlab param.vi"("Sampling frequency (Hz)"=w1606, "matlab wave file"=w1608, "index of AO wave"=w1611, "padding value"=w1610) -> ()  [unwired: 7 in]
                  }
                }
              }
              frame #3 {
                n4661 = case shown="True" w1614 {
                  tunnel: w1615 -> [_ w1622]
                  frame False {
                  }
                  frame True {
                    n4662 = local read "Meastab"() -> (w1619:enum32{"X-Y Image", "Linescan", "Timetrace"})
                    n4663 = call "waveformparamsv2.vi"("command"="get") -> ("Params out"=w1625:T16)  [unwired: 4 in, 2 out]
                    n4664 = Unbundle By Name(w1625) -> ("AO parameters"=w1624:T17)
                    n4665 = case shown="\"Timetrace\"" w1619 {
                      tunnel: [w1639 w1640] -> w1618
                      frame "X-Y Image", Default {
                        n4666 = local read "Sampling rate"() -> (w1639:dbl)
                      }
                      frame "Timetrace" {
                        n4667 = local read "srateAODOtt"() -> (w1640:dbl)
                      }
                    }
                    n4668 = Index Array(array=w1624, index=w1622) -> (element=w1623:T18)
                    n4669 = call "waveformsAObuffer.vi"("command"="get") -> ("AO wf out"=w1629:waveform(dbl)[])  [unwired: 1 in]
                    n4670 = call "matlabAOwffromparam.vi"("Cluster"=w1623) -> ("Waveform"=w1627:waveform(dbl))  [unwired: 1 out]
                    n4671 = property on="refwf" class="Ring (strict)"() -> ("RingText.Text"=w1630:string)  [unwired: 2 in, 2 out]
                    n4672 = Replace Array Subset(array=w1629, new element=w1627, index=w1622) -> (w1628:waveform(dbl)[])
                    n4673 = call "waveformsDObuffer.vi"("command"="get") -> ("DO wf out"=w1635:digitalwaveform[])  [unwired: 1 in]
                    n4674 = call "correctwaveformsizetemp.vi"("new sampling frequency (Hz)"=w1618, "start"=FALSE, "reference waveforms to"=w1630, "Analog waveforms in"=w1628, "stop"=FALSE, "Digital waveforms in"=w1635) -> ("analog wf out"=w1633:waveform(dbl)[], "Digital wf out"=w1631:digitalwaveform[], "measpoints"=w1620:i32)
                    n4675 = local read "wavdet"() -> (w1621:bool)
                    n4676 = local write "Analog Lines Plot"(w1633) -> ()
                    n4677 = call "GetNumCamFramesv2.vi"("Digital Waveform Graph"=w1631) -> ("Numeric"=w1632:i32)  [unwired: 10 in]
                    n4678 = local write "Digital Lines Plot"(w1631) -> ()
                    n4679 = call "waveformsAObuffer.vi"("AO wf in"=w1633, "command"="set") -> ()  [unwired: 1 out]
                    n4680 = call "waveformsDObuffer.vi"("DO wf in"=w1631, "command"="set") -> ()  [unwired: 1 out]
                    n4681 = local write "Total Camera Frames"(w1632) -> ()
                    n4682 = case shown="True" w1621 {
                      tunnel: w1620 -> [_ w1641]
                      frame False {
                      }
                      frame True {
                        n4683 = local write "# of frames"(w1641) -> ()
                      }
                    }
                  }
                }
              }
              frame #4 {
                n4684 = local read "finite samples"() -> (w1642:bool)
                n4685 = local read "continuous"() -> (w1643:bool)
                n4686 = local read "wavdet"() -> (w1644:bool)
                n4687 = call "2pparameters.vi"("command"="get") -> ("params out"=w1647:T12)  [unwired: 1 in]
                n4688 = Bundle By Name(cluster=w1647, "finite"=w1642, "cont"=w1643, "wavdet"=w1644) -> (w1645:T12)
                n4689 = call "2pparameters.vi"("Params in"=w1645, "command"="set") -> ()  [unwired: 1 out]
              }
            }
          }
          event "Load Matlab Waveform DO": Value Change {
            n4690 = event-data() -> ()  [unwired: 1 in, 6 out]
            n4691 = stacked-sequence {
              seq-local: [_ _ w1755 _ _] -> [_ _ _ w1770 _]
              seq-local: [_ _ w1754 _ _] -> [_ _ _ w1769 _]
              frame #0 {
                n4692 = local read "Measurement"() -> (w1649:T5)
                n4693 = case shown="\"X-Y-t movie\", Default" w1649 {
                  frame "X-Y-t movie", Default {
                    n4694 = local read "avpp"() -> (w1670:i32)
                    n4695 = local read "Angle ref"() -> (w1669:dbl)
                    n4696 = local read "ROI Type"() -> (w1668:u16)
                    n4697 = local read "xpixels ref"() -> (w1665:i32)
                    n4698 = local read "Vx-min ref"() -> (w1664:dbl)
                    n4699 = local read "Vx-max ref"() -> (w1663:dbl)
                    n4700 = local read "ypixels ref"() -> (w1661:i32)
                    n4701 = local read "Vy-min ref"() -> (w1662:dbl)
                    n4702 = local read "Vy-max ref"() -> (w1658:dbl)
                    n4703 = local read "Sampling rate"() -> (w1652:dbl)
                    n4704 = local read "finite samples"() -> (w1653:bool)
                    n4705 = local read "continuous"() -> (w1656:bool)
                    n4706 = local read "wavdet"() -> (w1657:bool)
                    n4707 = local read "# of frames"() -> (w1655:i32)
                    n4708 = local read "maxbufferAI"() -> (w1654:i32)
                    n4709 = local read "Override AI buffer"() -> (w1650:bool)
                    n4710 = call "2pparameters.vi"("command"="get") -> ("params out"=w1667:T12)  [unwired: 1 in]
                    n4711 = Bundle By Name(cluster=w1667, "type"="X-Y-t movie", "avpp"=w1670, "Angle Img"=w1669, "Xpixels Img"=w1665, "Vx-min Img"=w1664, "VX-max Img"=w1663, "Ypixels Img"=w1661, "Vy-min Img"=w1662, "Vy-max Img"=w1658, "srate"=w1652, "srate Img"=w1652, "finite"=w1653, "cont"=w1656, "wavdet"=w1657, "measpoints"=w1655, "maxbufferAI"=w1654, "Drawing Mode"=w1668, "Vz-reset"=0.0, "AIoverride"=w1650) -> (w1659:T12)
                    n4712 = call "2pparameters.vi"("Params in"=w1659, "command"="set") -> ()  [unwired: 1 out]
                  }
                  frame "X-Y-Z stack" {
                    n4713 = call "2pparameters.vi"("command"="get") -> ("params out"=w1674:T12)  [unwired: 1 in]
                    n4714 = Bundle By Name(cluster=w1674, "type"="X-Y-Z stack") -> (w1672:T12)
                    n4715 = call "2pparameters.vi"("Params in"=w1672, "command"="set") -> ()  [unwired: 1 out]
                  }
                  frame "Lifetime (scan)" {
                    n4716 = call "2pparameters.vi"("command"="get") -> ("params out"=w1679:T12)  [unwired: 1 in]
                    n4717 = Bundle By Name(cluster=w1679, "type"="Lifetime (scan)") -> (w1677:T12)
                    n4718 = call "2pparameters.vi"("Params in"=w1677, "command"="set") -> ()  [unwired: 1 out]
                  }
                  frame "Lifetime (contour)" {
                    n4719 = local read "Vy-min draw"() -> (w1689:dbl)
                    n4720 = local read "Vy-max draw"() -> (w1688:dbl)
                    n4721 = local read "Vx-min draw"() -> (w1691:dbl)
                    n4722 = local read "Vx-max draw"() -> (w1690:dbl)
                    n4723 = local read "xpixels ref"() -> (w1687:i32)
                    n4724 = local read "ypixels ref"() -> (w1686:i32)
                    n4725 = local read "ROI Type"() -> (w1685:u16)
                    n4726 = local read "srateAODOtt"() -> (w1696:dbl)
                    n4727 = local read "# of frames"() -> (w1701:i32)
                    n4728 = local read "refreshtime"() -> (w1693:dbl)
                    n4729 = local read "Pel"() -> (w1684:dbl)
                    n4730 = local read "bin"() -> (w1699:dbl)
                    n4731 = local read "Override AI buffer"() -> (w1682:bool)
                    n4732 = local read "finite samples"() -> (w1708:bool)
                    n4733 = local read "srateAODOtt"() -> (w1695:dbl)
                    n4734 = local read "srateAODOtt"() -> (w1702:dbl)
                    n4735 = local read "continuous"() -> (w1707:bool)
                    n4736 = local read "Angle ref"() -> (w1692:dbl)
                    n4737 = local read "wavdet"() -> (w1709:bool)
                    n4738 = local read "Vx-ref"() -> (w1704:dbl)
                    n4739 = local read "Vy-ref"() -> (w1706:dbl)
                    n4740 = local read "avpp"() -> (w1705:i32)
                    n4741 = call "tt_timeandsamples.vi"("bin"=w1699, "refreshtime"=w1693, "srateAODOtt"=w1696, "tot#ofsamples"=w1701) -> ("refreshrate"=w1697:dbl, "refreshbuffer"=w1698:i32, "timetracecycles"=w1703:i32)  [unwired: 5 in]
                    n4742 = local read "bin"() -> (w1700:dbl)
                    n4743 = call "2pparameters.vi"("command"="get") -> ("params out"=w1712:T12)  [unwired: 1 in]
                    n4744 = Bundle By Name(cluster=w1712, "Drawing Mode"=w1685, "measpoints"=w1701, "tt_cycles"=w1703, "refreshbuffer"=w1698, "refreshrate"=w1697, "Vx-ref"=w1704, "Vy-ref"=w1706, "srate"=w1695, "finite"=w1708, "cont"=w1707, "wavdet"=w1709, "avpp"=w1705, "srateAODO"=w1702, "bufferAI"=w1698, "bin"=w1700, "Angle Img"=w1692, "Vxminref"=w1691, "Vxmaxref"=w1690, "Vyminref"=w1689, "Vymaxref"=w1688, "Xpixels Img"=w1687, "Ypixels Img"=w1686, "Pel"=w1684, "Vz-reset"=0.0, "AIoverride"=w1682, "type"="Lifetime (contour)") -> (w1710:T12)
                    n4745 = Reciprocal(x=w1697) -> (1/x=w1694:dbl)
                    n4746 = local write "refreshtime"(w1694) -> ()
                    n4747 = call "2pparameters.vi"("Params in"=w1710, "command"="set") -> ()  [unwired: 1 out]
                  }
                  frame "X-Y-Z-t movie" {
                  }
                  frame "linescan" {
                  }
                  frame "Timetrace" {
                    n4748 = local read "Vy-min draw"() -> (w1722:dbl)
                    n4749 = local read "Vy-max draw"() -> (w1721:dbl)
                    n4750 = local read "Vx-min draw"() -> (w1724:dbl)
                    n4751 = local read "Vx-max draw"() -> (w1723:dbl)
                    n4752 = local read "xpixels ref"() -> (w1720:i32)
                    n4753 = local read "ypixels ref"() -> (w1719:i32)
                    n4754 = local read "ROI Type"() -> (w1718:u16)
                    n4755 = local read "srateAODOtt"() -> (w1729:dbl)
                    n4756 = local read "# of frames"() -> (w1734:i32)
                    n4757 = local read "refreshtime"() -> (w1726:dbl)
                    n4758 = local read "Pel"() -> (w1717:dbl)
                    n4759 = local read "bin"() -> (w1732:dbl)
                    n4760 = local read "Override AI buffer"() -> (w1715:bool)
                    n4761 = local read "finite samples"() -> (w1741:bool)
                    n4762 = local read "srateAODOtt"() -> (w1728:dbl)
                    n4763 = local read "srateAODOtt"() -> (w1735:dbl)
                    n4764 = local read "continuous"() -> (w1740:bool)
                    n4765 = local read "Angle ref"() -> (w1725:dbl)
                    n4766 = local read "wavdet"() -> (w1742:bool)
                    n4767 = local read "Vx-ref"() -> (w1737:dbl)
                    n4768 = local read "Vy-ref"() -> (w1739:dbl)
                    n4769 = local read "avpp"() -> (w1738:i32)
                    n4770 = call "tt_timeandsamples.vi"("bin"=w1732, "refreshtime"=w1726, "srateAODOtt"=w1729, "tot#ofsamples"=w1734) -> ("refreshrate"=w1730:dbl, "refreshbuffer"=w1731:i32, "timetracecycles"=w1736:i32)  [unwired: 5 in]
                    n4771 = local read "bin"() -> (w1733:dbl)
                    n4772 = call "2pparameters.vi"("command"="get") -> ("params out"=w1745:T12)  [unwired: 1 in]
                    n4773 = Bundle By Name(cluster=w1745, "Drawing Mode"=w1718, "measpoints"=w1734, "tt_cycles"=w1736, "refreshbuffer"=w1731, "refreshrate"=w1730, "Vx-ref"=w1737, "Vy-ref"=w1739, "srate"=w1728, "finite"=w1741, "cont"=w1740, "wavdet"=w1742, "avpp"=w1738, "srateAODO"=w1735, "bufferAI"=w1731, "bin"=w1733, "Angle Img"=w1725, "Vxminref"=w1724, "Vxmaxref"=w1723, "Vyminref"=w1722, "Vymaxref"=w1721, "Xpixels Img"=w1720, "Ypixels Img"=w1719, "Pel"=w1717, "Vz-reset"=0.0, "AIoverride"=w1715, "type"="Timetrace") -> (w1743:T12)
                    n4774 = Reciprocal(x=w1730) -> (1/x=w1727:dbl)
                    n4775 = local write "refreshtime"(w1727) -> ()
                    n4776 = call "2pparameters.vi"("Params in"=w1743, "command"="set") -> ()  [unwired: 1 out]
                  }
                  frame "Lifetime (point)" {
                  }
                }
              }
              frame #1 {
                w1748 = FALSE ("wavdet")
                n4777 = call "2pparameters.vi"("command"="get") -> ("params out"=w1752:T12)  [unwired: 1 in]
                n4778 = Bundle By Name(cluster=w1752, "finite"=w1748, "cont"=w1748, "wavdet"=TRUE) -> (w1749:T12)
                n4779 = call "2pparameters.vi"("Params in"=w1749, "command"="set") -> ()  [unwired: 1 out]
              }
              frame #2 {
                n4780 = local read "DO channels"() -> (w1757:u16)
                n4781 = call "2pparameters.vi"("command"="get") -> ("params out"=w1759:T12)  [unwired: 1 in]
                n4782 = Unbundle By Name(w1759) -> ("aDO"=w1758:u32[])
                n4783 = Search 1D Array(1D array=w1758, element=w1757) -> (index of element=w1755:i32)  [unwired: 1 in]
                n4784 = Greater?(x=w1755, y=-1) -> (0:w1754:bool)
                n4785 = case shown="True" w1754 {
                  tunnel: w1755 -> [_ w1766]
                  frame False {
                  }
                  frame True {
                    n4786 = local read "Meastab"() -> (w1762:enum32{"X-Y Image", "Linescan", "Timetrace"})
                    n4787 = local read "Matlab waveform path DO"() -> (w1764:path)
                    n4788 = local read "Matlab padding value DO"() -> (w1765:dbl)
                    n4789 = case shown="\"Timetrace\"" w1762 {
                      tunnel: [w1767 w1768] -> w1761
                      frame "X-Y Image", Default {
                        n4790 = local read "Sampling rate"() -> (w1767:dbl)
                      }
                      frame "Timetrace" {
                        n4791 = local read "srateAODOtt"() -> (w1768:dbl)
                      }
                    }
                    n4792 = call "matlabwfexistsdialogue.vi"("Matlab waveform path"=w1764) -> ("mtalab waveform path out"=w1763:path)
                    n4793 = call "replace DO matlab param.vi"("Sampling frequency (Hz)"=w1761, "matlab wave number"=w1763, "index of DO wave"=w1766, "padding value"=w1765) -> ()  [unwired: 7 in]
                  }
                }
              }
              frame #3 {
                n4794 = case shown="True" w1769 {
                  tunnel: w1770 -> [_ w1779]
                  frame False {
                  }
                  frame True {
                    n4795 = local read "Meastab"() -> (w1774:enum32{"X-Y Image", "Linescan", "Timetrace"})
                    n4796 = call "waveformparamsv2.vi"("command"="get") -> ("Params out"=w1792:T16)  [unwired: 4 in, 2 out]
                    n4797 = Unbundle By Name(w1792) -> ("DO parameters"=w1791:T19)
                    n4798 = case shown="\"Timetrace\"" w1774 {
                      tunnel: [w1794 w1795] -> w1773
                      frame "X-Y Image", Default {
                        n4799 = local read "Sampling rate"() -> (w1794:dbl)
                      }
                      frame "Timetrace" {
                        n4800 = local read "srateAODOtt"() -> (w1795:dbl)
                      }
                    }
                    n4801 = Index Array(array=w1791, index=w1779) -> (element=w1778:T20)
                    n4802 = call "waveformsDObuffer.vi"("command"="get") -> ("DO wf out"=w1789:digitalwaveform[])  [unwired: 1 in]
                    n4803 = property on="refwf" class="Ring (strict)"() -> ("RingText.Text"=w1781:string)  [unwired: 2 in, 2 out]
                    n4804 = call "matlabDOwffromparam.vi"("waveform params"=w1778) -> ("digital waveform"=w1777:digitalwaveform)
                    n4805 = Replace Array Subset(array=w1789, new element=w1777, index=w1779) -> (w1780:digitalwaveform[])
                    n4806 = call "waveformsAObuffer.vi"("command"="get") -> ("AO wf out"=w1788:waveform(dbl)[])  [unwired: 1 in]
